vi "SetReportingParameters.vi"(8 "error in":errorcluster, 10 "reporting parameters":T1[](array[typedef]), 11 "error reporter in":refnum<class "ErrorReporter.lvclass">) -> (0 "error out":errorcluster, 3 "error reporter out":refnum<class "ErrorReporter.lvclass">)   [LabVIEW 2013, in "CLM_ErrorHandler.lvlib" / "ErrorReporter.lvclass"]
uses:
  ErrorReporter.lvclass
  ReportingParameter.ctl
  ErrorReporter.lvclass/ErrorReporter.ctl
  Var_SetReportingParameter.vi
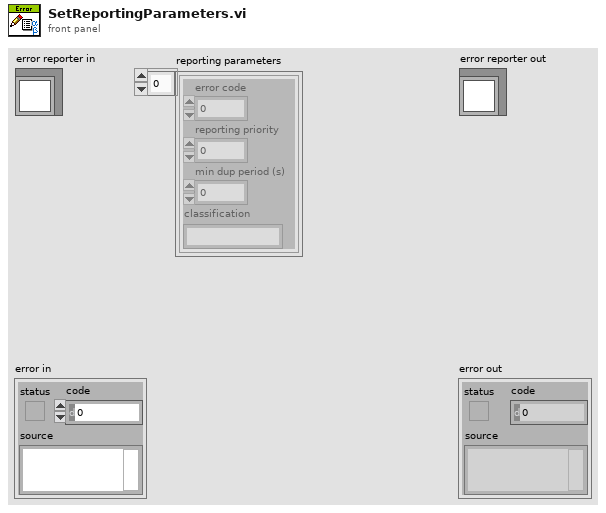
[diagram p1: front panel]
types:
  T1 = typedef "CLM_ErrorHandler.lvlib/ErrorReporter.lvclass/ReportingParameter.ctl" = cluster{"error code":i32, "reporting priority":i32, "min dup period (s)":dbl, "classification":string}
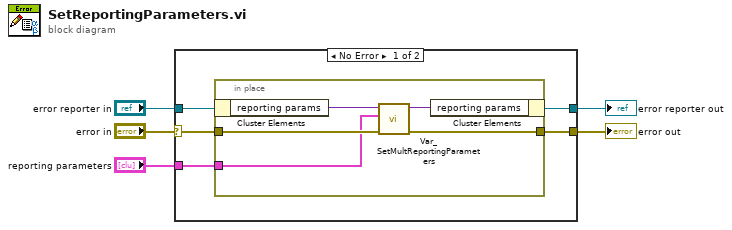
[diagram p0: block diagram]
diagram:
  n1 = case shown="No Error" "error in" {
    selector: "error in" -> [w7 w17]
    tunnel: [w8 w17] -> w4
    tunnel: [w9 w16] -> w2
    tunnel: "error reporter in" -> [w10 w16]
    tunnel: "reporting parameters" -> [w6 _]
    frame No Error {
      n2 = in-place {
        in-place-border: [w13] -> w8
        in-place-border: w7 -> [w12]
        in-place-border: w6 -> [w11]
        n3 = in-place-cluster #1(w10) -> ("reporting params"=w15:variant)
        n4 = call "Var_SetMultReportingParameters.vi"("error in"=w12, "reporting parameters"=w11, "reporting params in"=w15) -> ("error out"=w13:errorcluster, "reporting params out"=w14:variant)  [unwired: 6 in, 1 out]
        n5 = in-place-cluster #1("reporting params"=w14) -> (w9:refnum<class "ErrorReporter.lvclass">)
      }
    }
    frame Error {
    }
  }
  "error out" <- w4
  "error reporter out" <- w2
